vi "Load Parameters.vi"(8 "error in (no error)":errorcluster, 10 "Resource":variant, 11 "Analyze Actor in":refnum<class "Analyze Actor.lvclass">) -> (0 "error out":errorcluster, 3 "Analyze Actor out":refnum<class "Analyze Actor.lvclass">)   [LabVIEW 2020, in "Analyze Actor.lvlib" / "Analyze Actor.lvclass"]
uses:
  Analyze Actor.lvclass
  Analyze Actor.lvclass/Analyze Actor.ctl
  <vilib>/Utility/config.llb/NI_LVConfig.lvlib
  Analyze Classes/Analyze BaseClass/Analyze BaseClass/Analyze BaseClass.lvclass
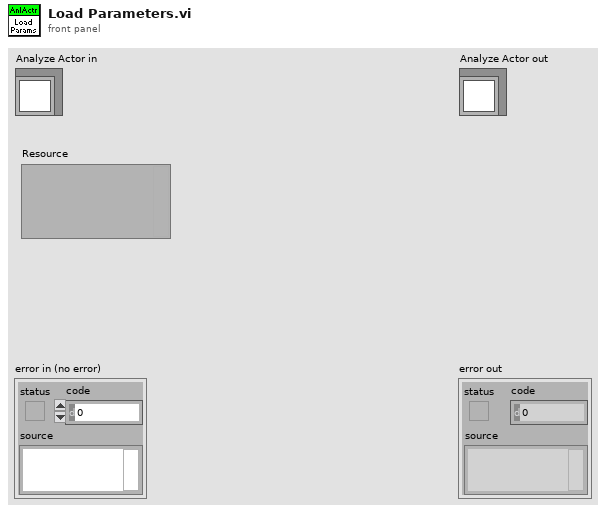
[diagram p1: front panel]
types:
  T1 = typedef "NI_LVConfig.lvlib/Config Data RefNum.ctl" = refnum<k1>
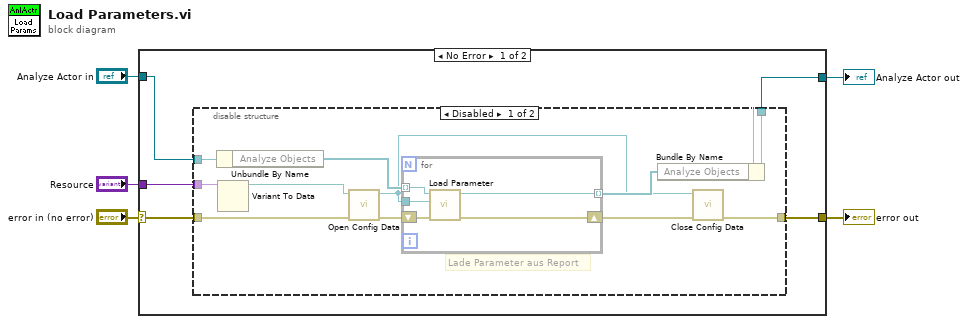
[diagram p0: block diagram]
diagram:
  n1 = case shown="No Error" "error in (no error)" {
    selector: "error in (no error)" -> [w8 w30]
    tunnel: [w7 w30] -> w4
    tunnel: [w9 w29] -> w2
    tunnel: "Analyze Actor in" -> [w10 w29]
    tunnel: "Resource" -> [w6 _]
    frame No Error {
      n2 = disable-structure shown="Disabled" {
        disable-tunnel: w10 -> [w21 w28]
        disable-tunnel: [w19 w28] -> w9
        disable-tunnel: w8 -> [w17 w27]
        disable-tunnel: [w14 w27] -> w7
        disable-tunnel: w6 -> [w13 _]
        frame Disabled {
          # "Lade Parameter aus Report"
          n3 = Unbundle By Name(w21) -> ("Analyze Objects"=w20:refnum<class "Analyze BaseClass.lvclass">[])
          n4 = Variant To Data(Variant=w13) -> (data=w12:path)  [unwired: 2 in, 1 out]
          n5 = call <vilib>:"Open Config Data.vi"("error in (no error)"=w17, "configuration file path"=w12) -> ("error out"=w16:errorcluster, "refnum"=w11:T1)  [unwired: 7 in, 1 out]
          n6 = for {
            tunnel: w20 -> [w26] mode=indexing
            tunnel: w11 -> [w25]
            shift-right: [w23] -> w15
            shift-left: w16 -> [w24]
            tunnel: [w22] -> w18 mode=indexing
            n7 = call-dynamic "Load Parameter.vi"("error in (no error)"=w24, "Resource"=w25, "Analyze BaseClass in"=w26) -> ("error out"=w23:errorcluster, "Analyze BaseClass out"=w22:refnum<class "Analyze BaseClass.lvclass">)  [unwired: 7 in]
          }
          n8 = Bundle By Name(cluster=w21, "Analyze Objects"=w18) -> (w19:refnum<class "Analyze Actor.lvclass">)
          n9 = call <vilib>:"Close Config Data.vi"("error in (no error)"=w15, "refnum"=w11) -> ("error out"=w14:errorcluster)  [unwired: 8 in, 1 out]
        }
        frame Enabled {
        }
      }
    }
    frame Error {
    }
  }
  "error out" <- w4
  "Analyze Actor out" <- w2
